vi "Create Counter Driven Output.vi"   [LabVIEW 2017, in "Scan Engine Scripting.lvlib"]
uses:
  Scan Engine Scripting.lvlib
  NI 9474/NI 9474.lvclass
  NI 9475/NI 9475.lvclass
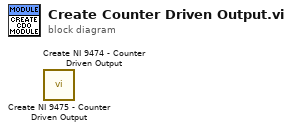
[diagram p0: block diagram]
diagram:
  n1 = call "Create NI 9475 - Counter Driven Output.vi"() -> ()  [unwired: 10 in, 2 out]
  n2 = call "Create NI 9474 - Counter Driven Output.vi"() -> ()  [unwired: 10 in, 2 out]
